vi "TTTR.vi"(0 "DeviceIndex":i32, 1 "Array":u8[](array[numeric]), 2 "file refnum":refnum<file>, 3 "error in (no error)":errorcluster) -> (4 "subarray":u8[](array[numeric]), 5 "OK":bool, 6 "FiFoOverrun":bool, 7 "error out":errorcluster, 8 "count":i32)   [LabVIEW 2013]
uses:
  phlib.dll
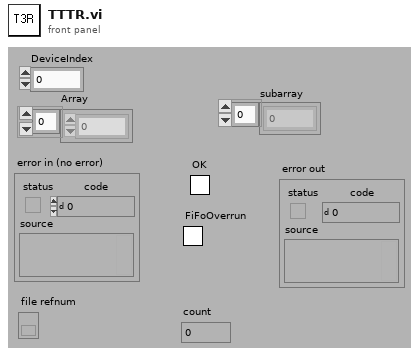
[diagram p1: front panel]
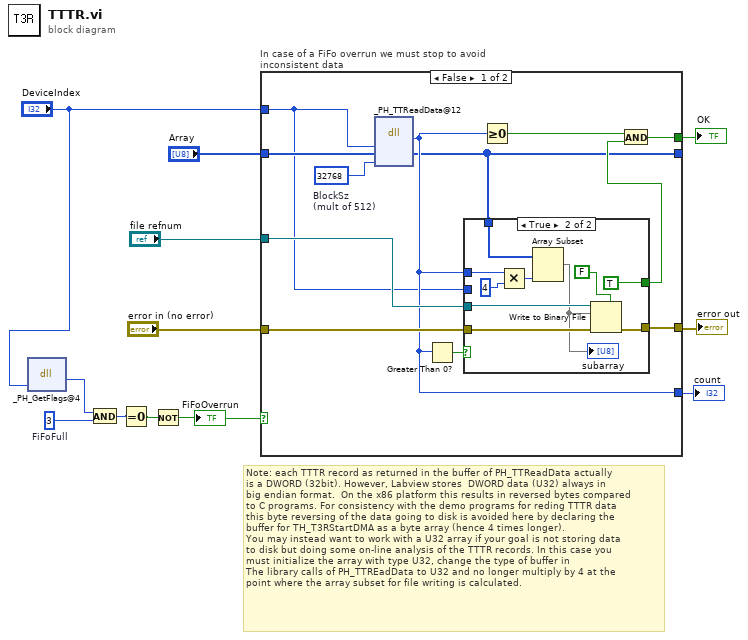
[diagram p0: block diagram]
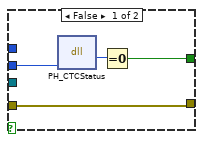
[diagram p2: hidden frame]
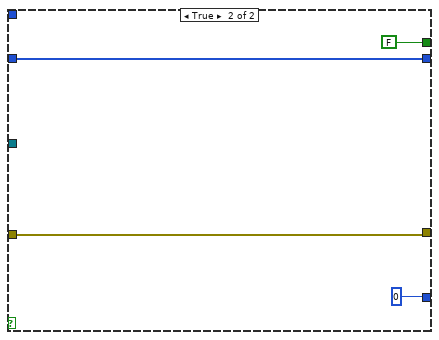
[diagram p3: hidden frame]
diagram:
  w7 = 3  # FiFoFull
  # "Note: each TTTR record as returned in the buffer of PH_TTReadData actually \nis a DWORD (32bit). However, Labview stores  DWORD data (U32) always in \nbig endian format.  On the x86 platform this results in reversed bytes compared \nto C programs. For consistency with the demo programs for reding TTTR data \nthis byte reversing of the data going to disk is avoided here by declaring the \nbuffer for TH_T3RStartDMA as a byte array (hence 4 times longer).\nYou may instead want to work with a U32 array if your goal is not storing data \nto disk but doing some on-line analysis of the TTTR records. In this case you \nmust initialize the array with type U32, change the type of buffer in\nThe library calls of PH_TTREadData to U32 and no longer multiply by 4 at the \npoint where the array subset for file writing is calculated."
  n1 = dll-call lib="phlib.dll" fn="_PH_GetFlags@4" label="PH_GetFlags"("devidx"="DeviceIndex") -> (w5:i32)  [unwired: 4 in, 2 out]
  n2 = And(x=w5, y=w7) -> (x .and. y?=w6:i32)
  n3 = Equal To 0?(x=w6) -> (x = 0?=w4:bool)
  n4 = Not ("CTCDone")(x=w4) -> (.not. x?=w3:bool)
  "FiFoOverrun" <- w3
  n5 = case "In case of a FiFo overrun we must stop to avoid inconsistent data" shown="False" w3 {
    tunnel: "Array" -> [w16 w41]
    tunnel: [w17 0] -> w12
    tunnel: [w15 w41] -> _
    tunnel: [w24 w40] -> w11
    tunnel: "error in (no error)" -> [w22 w40]
    tunnel: [w20 FALSE] -> w9
    tunnel: "file refnum" -> [w23 _]
    tunnel: "DeviceIndex" -> [w13 _]
    frame False {
      w14 = 32768  # BlockSz (mult of 512)
      n6 = dll-call lib="phlib.dll" fn="_PH_TTReadData@12" label="PH_TTReadData"("devidx"=w13, "buffer"=w16, "blocksize"=w14) -> (w17:i32, "buffer"=w15:u8[])  [unwired: 5 in, 2 out]
      n7 = Greater Than 0?(x=w17) -> (x > 0?=w21:bool)
      n8 = case shown="True" w21 {
        tunnel: [w28 w38] -> w24
        tunnel: w23 -> [_ w37]
        tunnel: w22 -> [w28 w36]
        tunnel: [w26 TRUE] -> w18
        tunnel: w15 -> [_ w34]
        tunnel: w17 -> [_ w32]
        tunnel: w13 -> [w25 _]
        frame False {
          n9 = dll-call lib="phlib.dll" fn="PH_CTCStatus"("devidx"=w25) -> (w27:i32)  [unwired: 4 in, 2 out]
          n10 = Equal To 0?(x=w27) -> (x = 0?=w26:bool)
        }
        frame True {
          n11 = Multiply(x=w32, y=4) -> (x*y=w33:i32)
          n12 = Array Subset(array=w34, length=w33) -> (w29:u8[])  [unwired: 1 in]
          "subarray" <- w29
          n13 = Write to Binary File(file (use dialog)=w37, data=w29, error in=w36, 5:FALSE ("prepend array or string size? (T)")) -> (error out=w38:errorcluster)  [unwired: 2 in, 2 out]
        }
      }
      n14 = Greater Or Equal To 0?(x=w17) -> (x >= 0?=w19:bool)
      n15 = And(x=w19, y=w18) -> (x .and. y?=w20:bool)
    }
    frame True {
    }
  }
  "OK" <- w9
  "count" <- w12
  "error out" <- w11
